vi "ReadAOs.vi"(8 "error in (no error)":errorcluster, 10 "Analog Output":T1, 11 "VISA resource name":refnum<visa-resource-name>) -> (0 "error out":errorcluster, 2 "AnOutValues":dbl[](array[numeric]), 3 "VISA resource name out":refnum<visa-resource-name>)   [LabVIEW 2020, in "HandsOnPi2040.lvlib"]
uses:
  <instrlib>/HandsOnPi2040/HandsOnPi2040.lvlib
  <instrlib>/HandsOnPi2040/Public/AOs.ctl
panel:
  out "read buffer":string
  # "Input"
  # "Output"
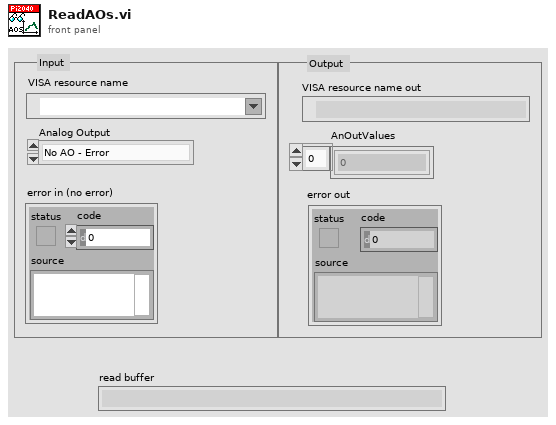
[diagram p1: front panel]
types:
  T1 = typedef "HandsOnPi2040.lvlib/AOs.ctl" = enum16{"No AO - Error", "AO1"}
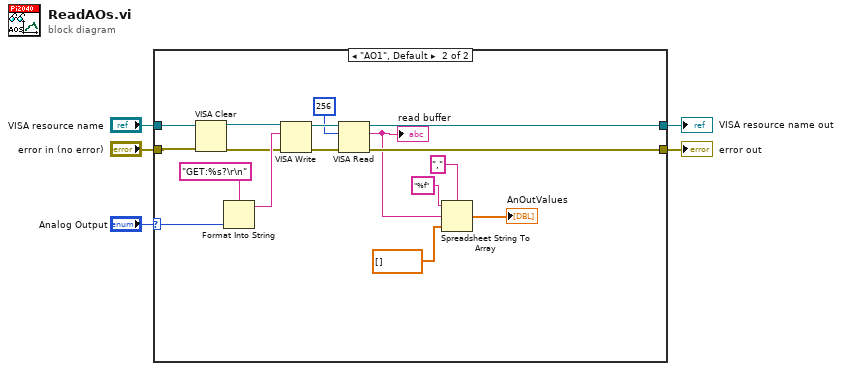
[diagram p0: block diagram]
diagram:
  n1 = case shown="\"AO1\", Default" "Analog Output" {
    selector: "Analog Output" -> [_ w17]
    tunnel: "VISA resource name" -> [w6 w11]
    tunnel: "error in (no error)" -> [w7 w10]
    tunnel: [w6 w19] -> w3
    tunnel: [w7 w18] -> w2
    frame "No AO - Error" {
    }
    frame "AO1", Default {
      n2 = VISA Clear(VISA resource name=w11, error in (no error)=w10) -> (VISA resource name out=w9:refnum<visa-resource-name>, error out=w8:errorcluster)
      n3 = Format Into String(format string="GET:%s?\r\n", w17) -> (resulting string=w20:string)  [unwired: 2 in, 1 out]
      n4 = VISA Write(VISA resource name=w9, write buffer=w20, error in (no error)=w8) -> (VISA resource name out=w23:refnum<visa-resource-name>, error out=w22:errorcluster)  [unwired: 1 out]
      n5 = VISA Read(VISA resource name=w23, byte count=u32 256, error in (no error)=w22) -> (VISA resource name out=w19:refnum<visa-resource-name>, read buffer=w15:string, error out=w18:errorcluster)  [unwired: 1 out]
      "read buffer" <- w15
      n6 = Spreadsheet String To Array(delimiter (Tab)=",", format string="%f", spreadsheet string=w15, array type (2D Dbl)=dbl[] [] ("AnOutValues")) -> (array=→"AnOutValues":dbl[])
    }
  }
  "VISA resource name out" <- w3
  "error out" <- w2
